vi "Analog Rotation Sensor.vi"(8 "reset angle":bool, 9 "invert direction":bool, 11 "Voltage":dbl) -> (1 "Rotations":dbl, 2 "Angle":dbl)   [LabVIEW 2012]
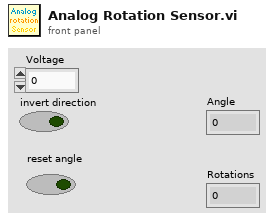
[diagram p1: front panel]
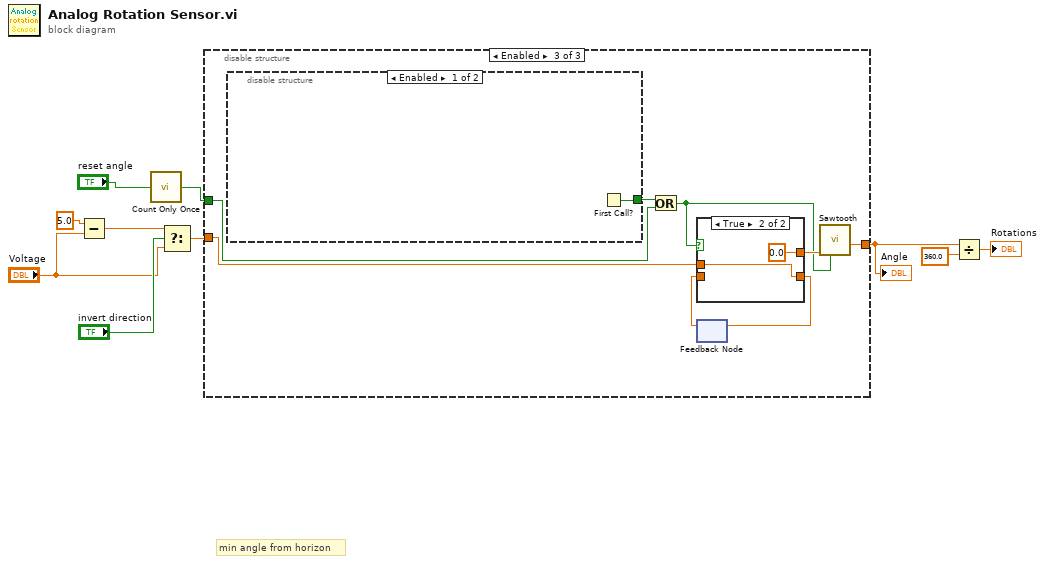
[diagram p0: block diagram]
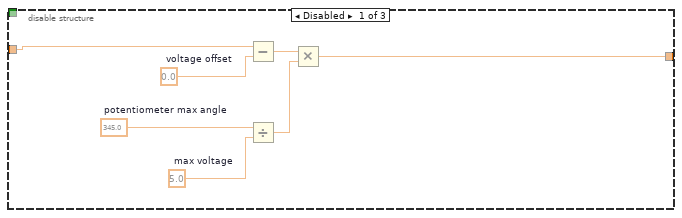
[diagram p2: hidden frame]
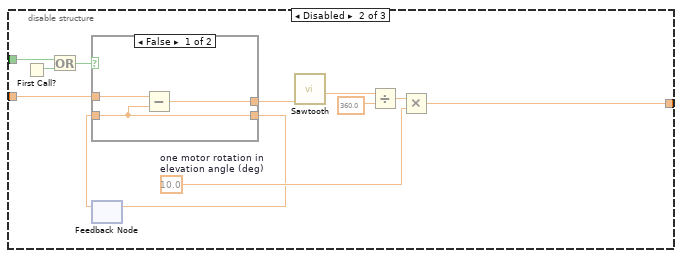
[diagram p3: hidden frame]
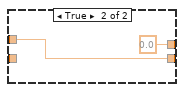
[diagram p4: hidden frame]
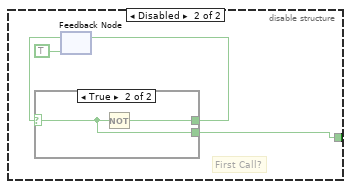
[diagram p5: hidden frame]
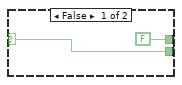
[diagram p6: hidden frame]
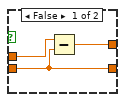
[diagram p7: hidden frame]
diagram:
  # "min angle from horizon"
  n1 = Subtract(x=5.0, y="Voltage") -> (x-y=w10:dbl)
  n2 = call "Count Only Once.vi"("InValue"="reset angle") -> ("Result"=w1:bool)
  n3 = Select(t=w10, s="invert direction", f="Voltage") -> (s? t:f=w8:dbl)
  n4 = disable-structure shown="Enabled" {
    disable-tunnel: w8 -> [w17 w25 w36]
    disable-tunnel: [w11 w18 w35] -> w5
    disable-tunnel: w1 -> [_ w20 w38]
    frame Disabled {
      w12 = 0.0  # voltage offset
      w15 = 5.0  # max voltage
      w16 = 345.0  # potentiometer max angle
      n5 = Subtract(x=w17, y=w12) -> (x-y=w13:dbl)
      n6 = Divide(x=w16, y=w15) -> (x/y=w14:dbl)
      n7 = Multiply(x=w13, y=w14) -> (x*y=w11:dbl)
    }
    frame Disabled {
      w26 = 10.0  # one motor rotation in elevation angle (deg)
      n8 = First Call?() -> (First Call?: T/F=w21:bool)
      n9 = Or(x=w20, y=w21) -> (x .or. y?=w19:bool)
      n10 = feedback #1() -> (w23:dbl)  [unwired: 1 in]
      n11 = case shown="False" w19 {
        tunnel: w25 -> [w32 w34]
        tunnel: [w31 w34] -> w24
        tunnel: w23 -> [w31 _]
        tunnel: [w30 0.0] -> w22
        frame False {
          n12 = Subtract(x=w32, y=w31) -> (x-y=w30:dbl)
        }
        frame True {
        }
      }
      n13 = feedback-in #1(w24) -> ()
      n14 = call "Sawtooth.vi"("Voltage"=w22) -> ("Absolute Angle (deg)"=w29:dbl)  [unwired: 8 in, 2 out]
      n15 = Divide(x=w29, y=360.0) -> (x/y=w27:dbl)
      n16 = Multiply(x=w27, y=w26) -> (x*y=w18:dbl)
    }
    frame Enabled {
      n17 = disable-structure shown="Enabled" {
        disable-tunnel: [w43 w45] -> w39
        frame Enabled {
          n18 = First Call?() -> (First Call?: T/F=w43:bool)
        }
        frame Disabled {
          # "First Call?"
          n19 = feedback #2(TRUE) -> (w47:bool)
          n20 = case shown="True" w47 {
            selector: w47 -> [w49 w51]
            tunnel: [w49 w51] -> w45
            tunnel: [FALSE w50] -> w44
            frame False {
            }
            frame True {
              n21 = Not(x=w51) -> (.not. x?=w50:bool)
            }
          }
          n22 = feedback-in #2(w44) -> ()
        }
      }
      n23 = Or(x=w39, y=w38) -> (x .or. y?=w37:bool)
      n24 = feedback #3() -> (w41:dbl)  [unwired: 1 in]
      n25 = case shown="True" w37 {
        tunnel: w36 -> [w54 w56]
        tunnel: [w53 w56] -> w42
        tunnel: w41 -> [w53 _]
        tunnel: [w52 0.0] -> w40
        frame False {
          n26 = Subtract(x=w54, y=w53) -> (x-y=w52:dbl)
        }
        frame True {
        }
      }
      n27 = feedback-in #3(w42) -> ()
      n28 = call "Sawtooth.vi"("Reintalize?"=w37, "Voltage"=w40) -> ("Absolute Angle (deg)"=w35:dbl)  [unwired: 7 in, 2 out]
    }
  }
  "Angle" <- w5
  n29 = Divide(x=w5, y=360.0) -> (x/y=→"Rotations":dbl)
